vi "Get UI VI Reference.vi"(8 "error in (no error)":errorcluster, 11 "Flex UI (Actor) in":refnum<class "Flex UI (Actor).lvclass">) -> (0 "error out":errorcluster, 2 "UI VI Reference":refnum<vi>, 3 "Flex UI (Actor) out":refnum<class "Flex UI (Actor).lvclass">)   [LabVIEW 2016, in "Flex UI (Parent Actor).lvlib" / "Flex UI (Actor).lvclass"]
uses:
  Flex UI (Actor).lvclass
  <vilib>/East West Architects/Flex UI/Flex UI (Parent)/Flex UI.lvclass
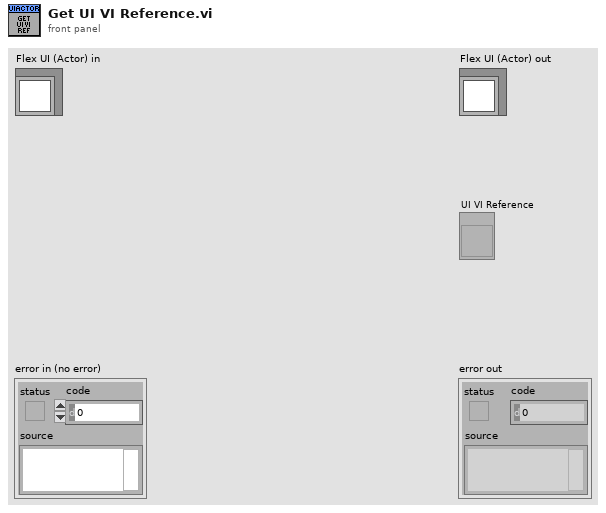
[diagram p1: front panel]
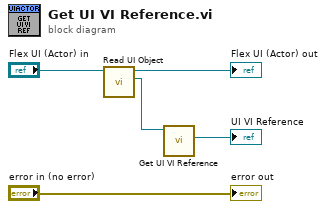
[diagram p0: block diagram]
diagram:
  n1 = call-dynamic "Read UI Object.vi"("Flex UI (Actor) in"="Flex UI (Actor) in") -> ("Flex UI Object"=w2:refnum<class "Flex UI.lvclass">, "Flex UI (Actor) out"=→"Flex UI (Actor) out":refnum<class "Flex UI (Actor).lvclass">)  [unwired: 8 in, 1 out]
  n2 = call-dynamic "Get UI VI Reference.vi"("Flex UI in"=w2) -> ("UI VI Reference"=→"UI VI Reference":refnum<vi>)  [unwired: 8 in, 2 out]
  "error out" <- "error in (no error)"
